vi "xlsKeithly_B1.vi"() -> ()   [LabVIEW 2012]
uses:
  Keithley 2600 Series/Keithley 2600 Series.lvlib
  Keithley 2600 Series/Public/Channel.ctl
  <vilib>/platform/TimedLoop/XDataNode/XDataNode.xnode
  <vilib>/Platform/TimedLoop/XDataNode/nitl_modes.ctl
  <vilib>/Platform/TimedLoop/XDataNode/XDNodeRunTimeDep.lvlib
  <vilib>/Platform/TimedLoop/XDataNode/wakeup.ctl
  <vilib>/Platform/TimedLoop/XDataNode/timing_clust.ctl
  <vilib>/Utility/file.llb/Write To Spreadsheet File (string).vi
  controls/KeithlyFunction.ctl
  controls/MeasurementType.ctl
  controls/KeithlyChannelType.ctl
panel:
  out "Current output of Channel A":dbl
  out "Current output of channel B":dbl
  out "Measurement chart A":cluster{dbl, "x+y":dbl}(graph)
  in  "Node":i8 min=0 max=64 step=1
  out "error out":errorcluster
  in  "Error Query (False)":bool
  in  "error in (no error)":errorcluster
  in  "VISA resource name":refnum<visa-resource-name>="GPIB0::26::INSTR"
  in  "ExitB":bool
  in  "StopB":bool
  in  "PlayB":bool
  in  "SaveB":bool
  out "Measurement chart B":cluster{dbl, "x+y":dbl}(graph)
  in  "ImportB":bool
  in  "Keithly functional input":T1[][](array[typedef])=[[{"Interval time"=10.0, "Input CH Type"=1, "Initial value"=0.0, "Final value"=5.0, "Sampling time"=0.1, "Meas. CH Type"=0}, {"Interval time"=10.0, "Input CH Type"=1, "Initial value"=0.0, "Final value"=10.0, "Sampling time"=0.1, "Meas. CH Type"=0}]] {"Meas. CH Type" items=["Current", "Voltage"]; "Input CH Type" items=["Current", "Voltage"]}
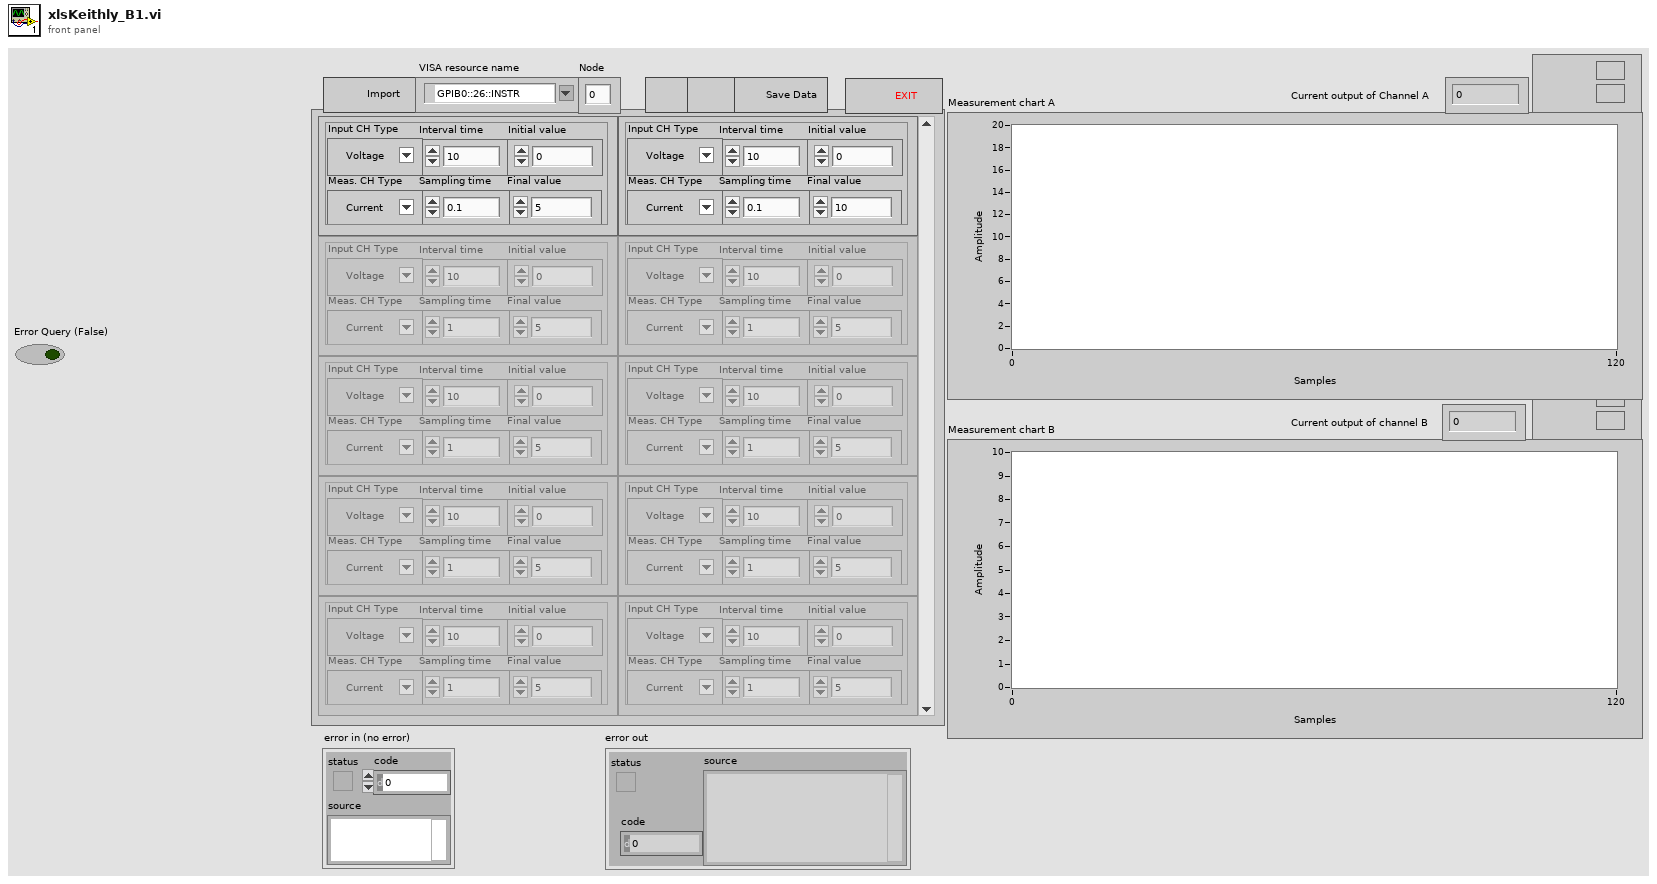
[diagram p1: front panel]
types:
  T1 = typedef "KeithlyFunction.ctl" = cluster{"Interval time":dbl, "Input CH Type":T2, "Initial value":dbl, "Final value":dbl, "Sampling time":dbl, "Meas. CH Type":T3}
  T2 = typedef "KeithlyChannelType.ctl" = u16
  T3 = typedef "MeasurementType.ctl" = u16
  T4 = typedef "XDNodeRunTimeDep.lvlib/timing_clust.ctl" = cluster{"Expected End [f-1]":u64, "Actual End [f-1]":u64, "Finished Late? [f-1]":bool, "Expected End [i-1]":u64, "Actual End [i-1]":u64, "Finished Late? [i-1]":bool, "Expected Start [i]":u64, "Actual Start [i]":u64, "Expected Start [f]":u64, "Actual Start [f]":u64, "Source Name":string, "Structure Name":string, "Period":i64, "Deadline":i64, "Offset":i64, "Start":i64, "Priority":i32, "Timeout":i32, "Mode":T5, "Wakeup Reason":T6, "Error":errorcluster, "Source Type":string, "Secondary Source Type":string, "Global End Time":u64, "Global Start Time":u64, "Frame Duration":u64, "Iteration Duration":u64, "Assigned CPU":i32, "I/O Scan Engine Mode":u32}
  T5 = typedef "XDNodeRunTimeDep.lvlib/nitl_modes.ctl" = enum32{"No Change", "Process missed periods, maintain original phase", "Discard missed periods, maintain original phase", "Process missed periods, ignore original phase", "Discard missed periods, ignore original phase"}
  T6 = typedef "XDNodeRunTimeDep.lvlib/wakeup.ctl" = enum32{"Normal", "Aborted", "Asynchronous wakeup", "Timing source error", "Timed loop error", "Timeout"}
  T7 = typedef "Keithley 2600 Series.lvlib/Channel.ctl" = enum32{"Channel A", "Channel B"}
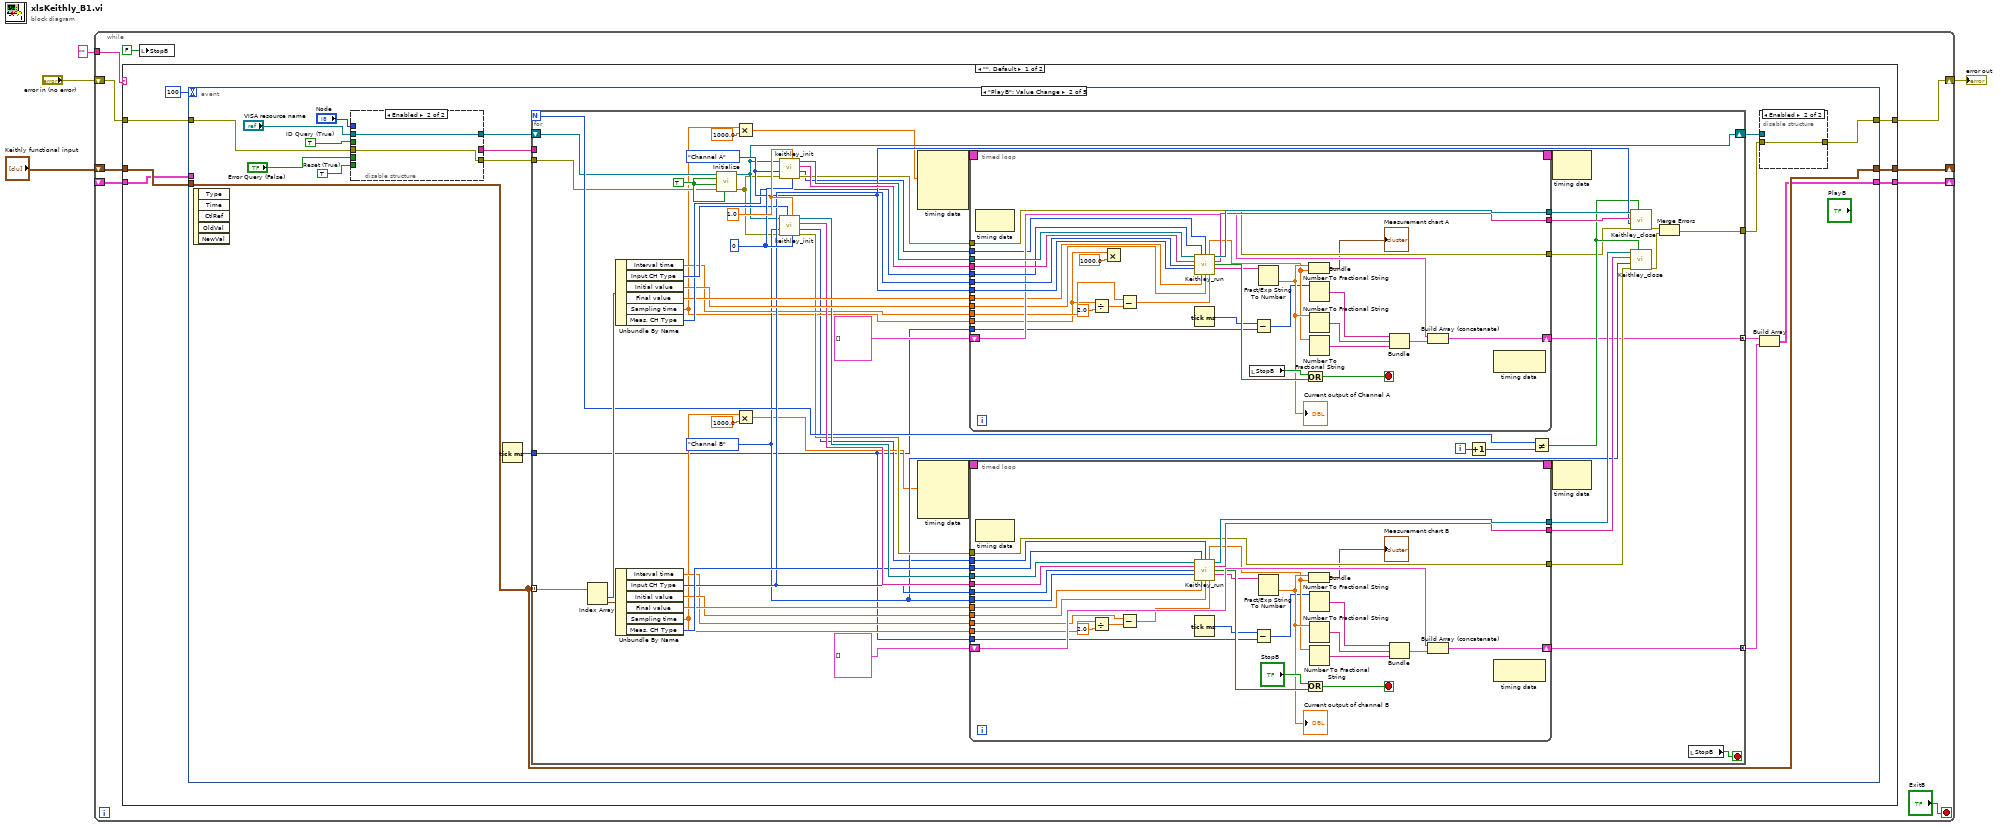
[diagram p0: block diagram]
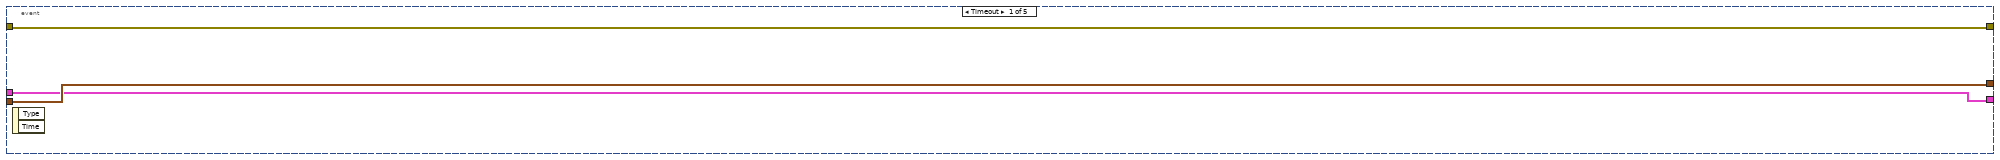
[diagram p2: hidden frame]
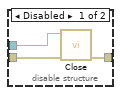
[diagram p3: hidden frame]
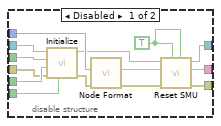
[diagram p4: hidden frame]
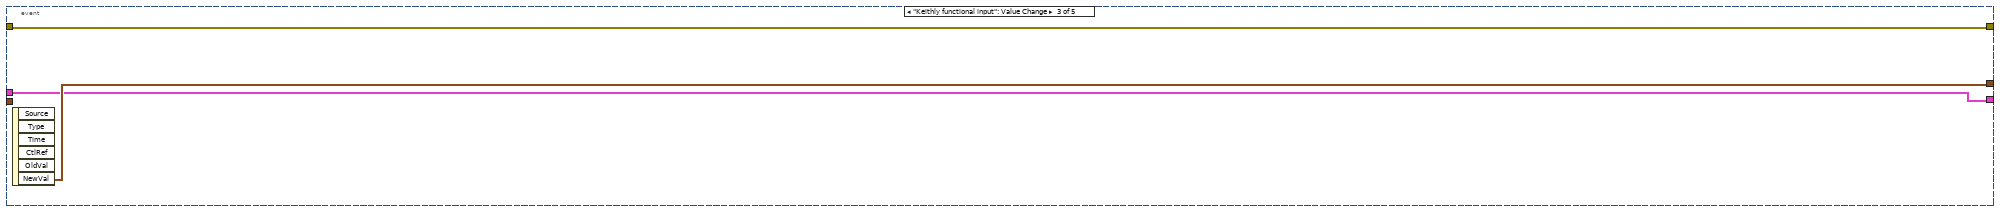
[diagram p5: hidden frame]
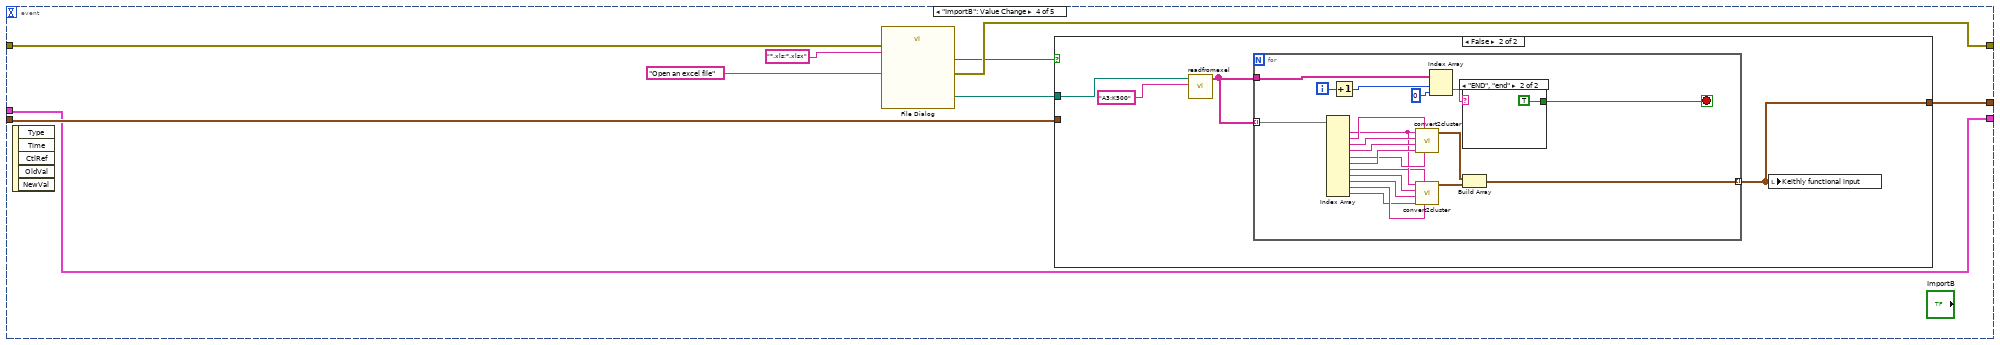
[diagram p6: hidden frame]
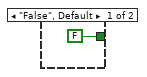
[diagram p8: hidden frame]
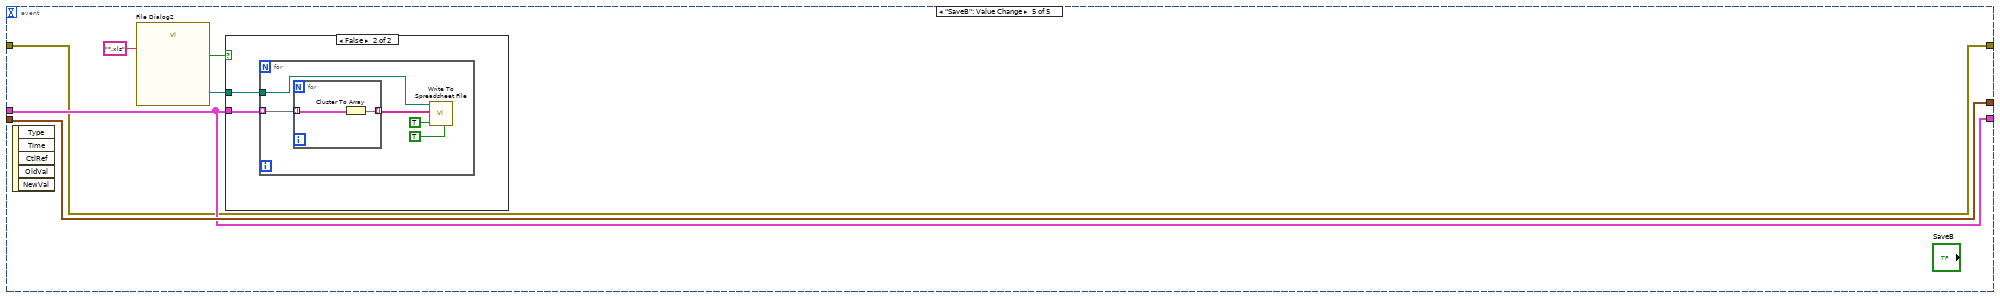
[diagram p9: hidden frame]
diagram:
  n1 = while {
    tunnel: "" -> [w12]
    shift-right: [w11] -> w3
    shift-left: "error in (no error)" -> [w10]
    shift-right: [w8] -> _
    shift-left: "Keithly functional input" -> [w9]
    shift-right: [w7] -> _
    shift-left: _ -> [w6]
    stop <- "ExitB" stop-if-true
    n2 = case shown="\"\", Default" w12 {
      tunnel: [w20 w254] -> w11
      tunnel: w10 -> [w19 w254]
      tunnel: w9 -> [w17 w253]
      tunnel: [w16 w253] -> w8
      tunnel: [w15 w252] -> w7
      tunnel: w6 -> [w14 w252]
      frame "", Default {
        n3 = event shown="[1] \"PlayB\": Value Change" {
          selector: _ -> [_ _ _ _ _]
          dyn-events: _ -> [_ _ _ _ _]
          timeout: 100 -> [_ _ _ _ _]
          tunnel: [w21 w30 w198 w206 w237] -> w20
          tunnel: w19 -> [w21 w29 w198 w207 w237]
          tunnel: w17 -> [w23 w28 _ w201 w240]
          tunnel: [w23 w28 w199 w202 w240] -> w16
          tunnel: [w22 w27 w197 w200 w238] -> w15
          tunnel: w14 -> [w22 _ w197 w200 w238]
          event Timeout {
            n4 = event-data() -> ()  [unwired: 1 in, 2 out]
          }
          event "PlayB": Value Change {
            w39 = TRUE  # Reset (True)
            w32 = TRUE  # ID Query (True)
            n5 = event-data() -> ()  [unwired: 1 in, 5 out]
            n6 = disable-structure shown="Enabled" {
              disable-tunnel: "Node" -> [w58 _]
              disable-tunnel: w39 -> [w54 _]
              disable-tunnel: [w53 _] -> w36
              disable-tunnel: [w52 w59] -> w35
              disable-tunnel: [w51 w60] -> w34
              disable-tunnel: "Error Query (False)" -> [w49 _]
              disable-tunnel: w32 -> [w48 _]
              disable-tunnel: "VISA resource name" -> [w47 w59]
              disable-tunnel: w29 -> [w46 w60]
              frame Disabled {
                w45 = TRUE ("SMU B (No)")
                n7 = call "Initialize.vi"("Reset (True)"=w54, "error in (no error)"=w46, "Error Query (False)"=w49, "ID Query (True)"=w48, "VISA resource name"=w47) -> ("error out"=w56:errorcluster, "VISA resource name out"=w50:refnum<visa-resource-name>)  [unwired: 1 in, 4 out]
                n8 = call "Node Format.vi"("error in"=w56, "Node (0-64)"=w58) -> ("error out"=w57:errorcluster, "Formatted Node"=w55:string)  [unwired: 8 out]
                n9 = call "Reset SMU.vi"("SMU B (No)"=w45, "SMU A (No)"=w45, "error in (no error)"=w57, "Node In"=w55, "VISA resource name"=w50) -> ("error out"=w51:errorcluster, "Node Out"=w53:string, "VISA resource name out"=w52:refnum<visa-resource-name>)  [unwired: 4 out]
              }
              frame Enabled {
              }
            }
            n10 = Tick Count (ms)() -> (millisecond timer value=w24:u32)
            n11 = for {
              N -> [w91]
              tunnel: [w116] -> w37
              tunnel: w36 -> [_]
              tunnel: w34 -> [w85]
              shift-right: [w83] -> w38
              shift-left: w35 -> [w84]
              tunnel: w28 -> [w119] mode=indexing
              tunnel: [w77] -> w26 mode=concatenating
              tunnel: [w76] -> w25 mode=concatenating
              tunnel: w24 -> [w61]
              i -> [w92]
              stop <- w93 stop-if-true
              w115 = 1.0 ("Limit in")
              w114 = i8 0 ("Node (0-64) in")
              w86 = TRUE ("Error Query (False) in")
              w107 = Channel."Channel A" ("Channel (Channel A)")
              w82 = Channel."Channel B" ("Channel (Channel A) 2")
              n12 = Index Array(array=w119) -> (element #1=w118:T1, element #2=w117:T1)  [unwired: 2 in]
              n13 = Unbundle By Name(w118) -> ("Interval time"=w94:dbl, "Input CH Type"=w108:T2, "Initial value"=w104:dbl, "Final value"=w105:dbl, "Sampling time"=w71:dbl, "Meas. CH Type"=w106:T3)
              n14 = Unbundle By Name(w117) -> ("Interval time"=w95:dbl, "Input CH Type"=w98:T2, "Initial value"=w96:dbl, "Final value"=w97:dbl, "Sampling time"=w65:dbl, "Meas. CH Type"=w99:T3)
              n15 = call "Initialize.vi"("Reset (True)"=w86, "error in (no error)"=w85, "Error Query (False)"=w86, "ID Query (True)"=w86, "VISA resource name"=w84) -> ("error out"=w81:errorcluster, "VISA resource name out"=w83:refnum<visa-resource-name>)  [unwired: 1 in, 4 out]
              n16 = Multiply(x=w71, y=1000.0) -> (x*y=w70:dbl)
              n17 = Multiply(x=w65, y=1000.0) -> (x*y=w66:dbl)
              n18 = call "keithley_init.vi"("Node (0-64) in"=w114, "Limit in"=w115, "error in (no error)"=w81, "Channel (Channel A) in"=w107, "VISA Refnum in"=w83) -> ("error out"=w80:errorcluster, "Init timer"=w64:u32, "Node Out"=w109:string, "VISA resource name out"=w112:refnum<visa-resource-name>)  [unwired: 3 in]
              n19 = call "keithley_init.vi"("Node (0-64) in"=w114, "Limit in"=w115, "Source Function (Current) 3"=w98, "error in (no error)"=w81, "Channel (Channel A) in"=w82, "VISA Refnum in"=w83) -> ("error out"=w88:errorcluster, "Init timer"=w63:u32, "Node Out"=w100:string, "VISA resource name out"=w101:refnum<visa-resource-name>)  [unwired: 2 in]
              n20 = node-c288(w70) -> (w74:T4)  [unwired: 3 in]
              n21 = node-c288(w66) -> (w68:T4)  [unwired: 3 in]
              n22 = timed-loop {
                tunnel: w112 -> [w190]
                tunnel: [w189] -> w111
                tunnel: [w188] -> w110
                tunnel: w109 -> [w187]
                tunnel: w108 -> [w186]
                tunnel: w107 -> [w185]
                tunnel: w106 -> [w184]
                shift-right: [w183] -> w76
                shift-left: cluster{string, string, string}[] [] -> [w182]
                tunnel: w94 -> [w180]
                tunnel: w71 -> [w159]
                tunnel: w105 -> [w181]
                tunnel: w104 -> [w179]
                tunnel: w64 -> [w178]
                tunnel: w80 -> [w172]
                tunnel: [w172] -> w79
                tunnel: w61 -> [w169]
                timing: w74 -> [_]
                timing-out: [_] -> w73
                stop <- w176 stop-if-true
                n23 = node-c288() -> ()  [unwired: 1 in, 1 out]
                n24 = Divide(x=w159, y=2.0) -> (x/y=w160:dbl)
                n25 = Multiply(x=w159, y=1000.0) -> ()  [unwired: 1 out]
                n26 = Subtract(x=w180, y=w160) -> (x-y=w161:dbl)
                n27 = call "Keithley_run.vi"("VISA Refnum in"=w190, "Meas. CH Type"=w184, "Init timer"=w178, "Node Out"=w187, "Input CH Type"=w186, "Channel (Channel A)"=w185, "Final value"=w181, "Initial value"=w179, "Interval time"=w161) -> ("x+y"=w165:dbl, "VISA Refnum out"=w189:refnum<visa-resource-name>, "Node Out out"=w188:string, "Boolean"=w175:bool, "Output"=w173:string)  [unwired: 1 in, 1 out]
                n28 = Tick Count (ms)() -> (millisecond timer value=w170:u32)
                n29 = local read "StopB"() -> (w177:bool)
                n30 = Subtract(x=w170, y=w169) -> (x-y=w163:u32)
                n31 = Fract/Exp String To Number(string=w173) -> (number=w166:dbl)  [unwired: 3 in, 1 out]
                "Current output of Channel A" <- w166
                n32 = Or(x=w177, y=w175) -> (x .or. y?=w176:bool)
                n33 = Bundle(w166, "x+y"=w165) -> (→"Measurement chart A":cluster{dbl, "x+y":dbl})  [unwired: 1 in]
                n34 = Number To Fractional String(number=w163) -> (F-format string=w164:string)  [unwired: 3 in]
                n35 = Number To Fractional String(number=w166) -> (F-format string=w171:string)  [unwired: 3 in]
                n36 = Number To Fractional String(number=w165) -> (F-format string=w168:string)  [unwired: 3 in]
                n37 = Bundle(w164, w171, w168) -> (w162:cluster{string, string, string})  [unwired: 1 in]
                n38 = Build Array (concatenate)(w182, w162) -> (w183:cluster{string, string, string}[])
                n39 = node-c288() -> ()  [unwired: 1 in, 1 out]
              }
              n40 = timed-loop {
                tunnel: w101 -> [w151]
                tunnel: [w150] -> w103
                tunnel: [w149] -> w102
                tunnel: w100 -> [w148]
                shift-right: [w147] -> w77
                shift-left: cluster{string, string, string}[] [] -> [w146]
                tunnel: w63 -> [w145]
                tunnel: w99 -> [w144]
                tunnel: w98 -> [w143]
                tunnel: w82 -> [w142]
                tunnel: w97 -> [w141]
                tunnel: w96 -> [w140]
                tunnel: w95 -> [w123]
                tunnel: w65 -> [w121]
                tunnel: w88 -> [w136]
                tunnel: [w136] -> w87
                tunnel: w61 -> [w132]
                timing: w68 -> [_]
                timing-out: [_] -> w67
                stop <- w137 stop-if-true
                n41 = node-c288() -> ()  [unwired: 1 in, 1 out]
                n42 = Divide(x=w121, y=2.0) -> (x/y=w122:dbl)
                n43 = Subtract(x=w123, y=w122) -> (x-y=w124:dbl)
                n44 = call "Keithley_run.vi"("VISA Refnum in"=w151, "Meas. CH Type"=w144, "Init timer"=w145, "Node Out"=w148, "Input CH Type"=w143, "Channel (Channel A)"=w142, "Final value"=w141, "Initial value"=w140, "Interval time"=w124) -> ("x+y"=w128:dbl, "VISA Refnum out"=w150:refnum<visa-resource-name>, "Node Out out"=w149:string, "Boolean"=w138:bool, "Output"=w134:string)  [unwired: 1 in, 1 out]
                n45 = Tick Count (ms)() -> (millisecond timer value=w133:u32)
                n46 = Subtract(x=w133, y=w132) -> (x-y=w125:u32)
                n47 = Fract/Exp String To Number(string=w134) -> (number=w129:dbl)  [unwired: 3 in, 1 out]
                "Current output of channel B" <- w129
                n48 = Or(x="StopB", y=w138) -> (x .or. y?=w137:bool)
                n49 = Bundle(w129, "x+y"=w128) -> (→"Measurement chart B":cluster{dbl, "x+y":dbl})  [unwired: 1 in]
                n50 = Number To Fractional String(number=w125) -> (F-format string=w126:string)  [unwired: 3 in]
                n51 = Number To Fractional String(number=w129) -> (F-format string=w135:string)  [unwired: 3 in]
                n52 = Number To Fractional String(number=w128) -> (F-format string=w131:string)  [unwired: 3 in]
                n53 = Bundle(w126, w135, w131) -> (w127:cluster{string, string, string})  [unwired: 1 in]
                n54 = Build Array (concatenate)(w146, w127) -> (w147:cluster{string, string, string}[])
                n55 = node-c288() -> ()  [unwired: 1 in, 1 out]
              }
              n56 = Increment(x=w92) -> (x+1=w90:i32)
              n57 = Not Equal?(x=w91, y=w90) -> (x != y?=w89:bool)
              n58 = node-c288(w73) -> ()  [unwired: 1 out]
              n59 = node-c288(w67) -> ()  [unwired: 1 out]
              n60 = call "Keithley_close.vi"("enable"=w89, "error in (no error)"=w79, "Channel (Channel A) in"=w107, "Node Out"=w110, "VISA Refnum in"=w111) -> ("error out"=w113:errorcluster)  [unwired: 6 in]
              n61 = call "Keithley_close.vi"("enable"=w89, "error in (no error)"=w87, "Channel (Channel A) in"=w82, "Node Out"=w102, "VISA Refnum in"=w103) -> ("error out"=w78:errorcluster)  [unwired: 6 in]
              n62 = Merge Errors(w113, w78) -> (w116:errorcluster)
              n63 = local read "StopB"() -> (w93:bool)
            }
            n64 = disable-structure shown="Enabled" {
              disable-tunnel: w38 -> [w43 _]
              disable-tunnel: w37 -> [w42 w44]
              disable-tunnel: [w41 w44] -> w30
              frame Disabled {
                n65 = call "Close.vi"("error in (no error)"=w42, "VISA resource name"=w43) -> ("error out"=w41:errorcluster)  [unwired: 9 out]
              }
              frame Enabled {
              }
            }
            n66 = Build Array(w25, w26) -> (w27:cluster{string, string, string}[][])
          }
          event "Keithly functional input": Value Change {
            n67 = event-data() -> ("NewVal"=w199:T1[][])  [unwired: 1 in, 5 out]
          }
          event "ImportB": Value Change {
            n68 = event-data() -> ()  [unwired: 1 in, 5 out]
            n69 = call "File Dialog"("prompt"="Open an excel file", "error in"=w207, "pattern (all files)"="*.xls;*.xlsx") -> ("selected path"=w208:path, "cancelled"=w203:bool, "error out"=w206:errorcluster)  [unwired: 9 in, 1 out]
            n70 = case shown="False" w203 {
              tunnel: w208 -> [_ w213]
              tunnel: [w209 w211] -> w202
              tunnel: w201 -> [w209 _]
              frame True {
              }
              frame False {
                n71 = call "readfromexel.vi"("RANGE"="A3:K500", "Path"=w213) -> ("Element 1"=w210:string[][])  [unwired: 7 in]
                n72 = for {
                  tunnel: w210 -> [w234] mode=indexing
                  tunnel: [w226] -> w211 mode=indexing
                  tunnel: w210 -> [w225]
                  i -> [w224]
                  stop <- w220 stop-if-true
                  n73 = Index Array(array=w234) -> (element #1=w219:string, element #2=w229:string, element #3=w233:string, element #4=w232:string, element #5=w230:string, element #6=w231:string, element #7=w218:string, element #8=w217:string, element #9=w216:string, element #10=w215:string, element #11=w214:string)  [unwired: 11 in]
                  n74 = Increment(x=w224) -> (x+1=w222:i32)
                  n75 = call "convert2cluster.vi"("Measurement CH type"=w230, "Input CH type"=w229, "Sampling time"=w231, "Final value"=w232, "Initial value"=w233, "Interval time"=w219) -> ("element"=w228:T1)  [unwired: 5 in]
                  n76 = call "convert2cluster.vi"("Measurement CH type"=w215, "Input CH type"=w218, "Sampling time"=w214, "Final value"=w216, "Initial value"=w217, "Interval time"=w219) -> ("element"=w227:T1)  [unwired: 5 in]
                  n77 = Index Array(array=w225, index (row)=w222, index (col)=0 ("disabled index (col)")) -> (element=w221:string)
                  n78 = case shown="\"END\", \"end\"" w221 {
                    tunnel: [FALSE TRUE] -> w220
                    frame "False", Default {
                    }
                    frame "END", "end" {
                    }
                  }
                  n79 = Build Array(w228, w227) -> (w226:T1[])
                }
                n80 = local write "Keithly functional input"(w211) -> ()
              }
            }
          }
          event "SaveB": Value Change {
            n81 = event-data() -> ()  [unwired: 1 in, 5 out]
            n82 = call "File Dialog2"("pattern (all files)"="*.xls") -> ("selected path"=w239:path, "cancelled"=w241:bool)  [unwired: 11 in, 2 out]
            n83 = case shown="False" w241 {
              tunnel: w239 -> [_ w244]
              tunnel: w238 -> [_ w243]
              frame True {
              }
              frame False {
                n84 = for {
                  tunnel: w244 -> [w249]
                  tunnel: w243 -> [w247] mode=indexing
                  n85 = for {
                    tunnel: w247 -> [w251] mode=indexing
                    tunnel: [w250] -> w246 mode=indexing
                    n86 = Cluster To Array(cluster=w251) -> (array=w250:string[])
                  }
                  n87 = call-poly <vilib>:"Write To Spreadsheet File.vi"("transpose? (no:F)"=TRUE, "append to file? (new file:F)"=TRUE, "2D data"=w246, "file path (dialog if empty)"=w249) -> ()  [unwired: 4 in, 1 out]
                }
              }
            }
          }
        }
      }
      frame "True" {
      }
    }
    n88 = local write "StopB"(FALSE ("StopB")) -> ()
  }
  "error out" <- w3
